vi "GetTerms3.vi"(0 "XRef":T10, 1 "State In":T9) -> (14 "Terms":T1)   [LabVIEW 2012, in "OpenG Search Array.xnode"]
doc: "This ability VI is used to describe your terminals to LabVIEW. Terms is an array of clusters describing the XNode's terminals.\n ID: A unique string identifying the terminal.\n Name: The name of the terminal visible to the user. Remember to localize it.\n Type: The data type of the terminal (as a Variant). The data put in the variant will be used as the default for the input terminal if it's left unwired.\n Bounds: A rectangle defining the bounds of the terminal relative to the bounds of the XNode. The bounds must be within the bounds of the XNode, and for whiskers to draw properly, they must be flush with at least one side of the XNode.\n Input?: Indicates whether or not this terminals is an input.\n Required?: Indicates whether the user must wire this terminal for the XNode to not be broken. Ignored on outputs.\n Recommended?: Indicates whether the terminal is recommended.\n Hidden?: Indicates whether the terminal is hidden. When a terminal is hidden, it cannot be wired to via user interaction or scripting. However, if it is already wired to when the hidden flag is changed to true, it will remain wired.\n Adaptive?: Indicates that the term should change to match the type of its source if it is wired.\n Direction?: Indicates what direction the wire stub should point. Choose auto to let LV decide based on the terms bounds being on the nodes edge.\n \n The IDs are used by LabVIEW to keep track of your terminals. When you respecify your terminals, LabVIEW can tell whther terminals are new, deleted, or moved by the unique IDs. The order is irrelevant. If you move a terminal, then any wire connected to it will move with it.\n \n If you want to update your terminals, you should return the UpdateTerms reply in one of your ability VIs.\n\nDefault behavior: None.\n\nThis ability does not provide UI and OS messages are not handled."
uses:
  OpenG Search Array.xnode
  <vilib>/XNodeSupport/XNodeXNodeRef.ctl
  State.ctl
  <vilib>/XNodeSupport/XNodeTerm3Array.ctl
  <vilib>/XNodeSupport/XNodeTerm3.ctl
  <vilib>/XNodeSupport/XNodeString.ctl
  <vilib>/XNodeSupport/XNodeVariant.ctl
  <vilib>/XNodeSupport/XNodeRect32.ctl
  <vilib>/XNodeSupport/XNodeInt.ctl
  <vilib>/XNodeSupport/XNodeBool.ctl
  <vilib>/XNodeSupport/XNodeTermDirection.ctl
  <vilib>/XNodeSupport/NI_XNodeSupport.lvlib
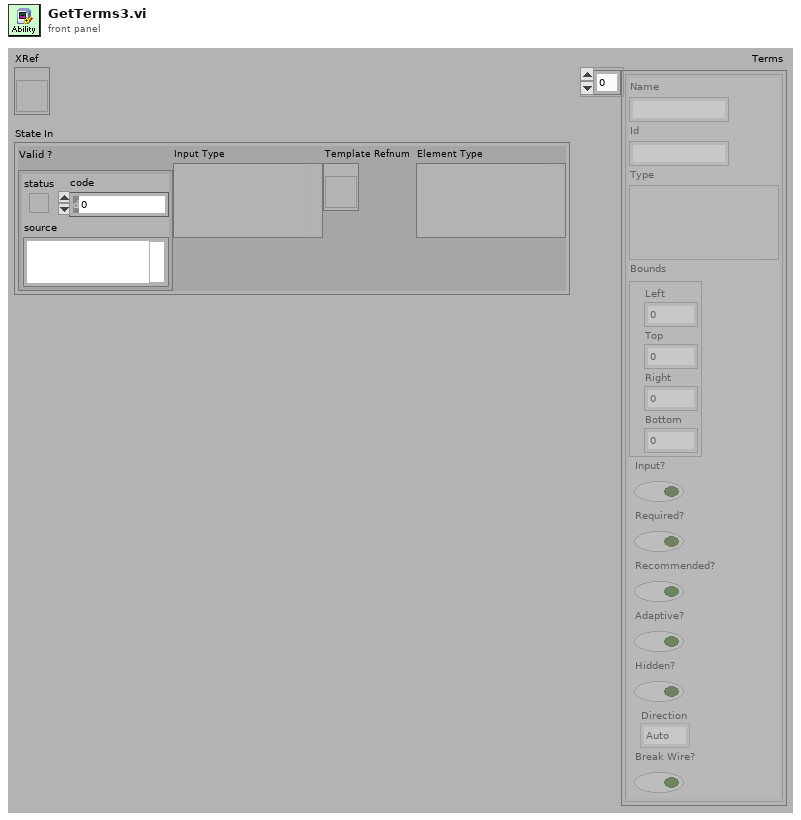
[diagram p1: front panel]
types:
  T1 = typedef "NI_XNodeSupport.lvlib/XNodeTerm3Array.ctl" = T2[]
  T2 = typedef "NI_XNodeSupport.lvlib/XNodeTerm3.ctl" = cluster{"Name":T3, "Id":T3, "Type":T4, "Bounds":T5, "Input?":T7, "Required?":T7, "Recommended?":T7, "Adaptive?":T7, "Hidden?":T7, "Direction":T8, "Break Wire?":T7}
  T3 = typedef "NI_XNodeSupport.lvlib/XNodeString.ctl" = string
  T4 = typedef "NI_XNodeSupport.lvlib/XNodeVariant.ctl" = variant
  T5 = typedef "NI_XNodeSupport.lvlib/XNodeRect32.ctl" = cluster{"Left":T6, "Top":T6, "Right":T6, "Bottom":T6}
  T6 = typedef "NI_XNodeSupport.lvlib/XNodeInt.ctl" = i32
  T7 = typedef "NI_XNodeSupport.lvlib/XNodeBool.ctl" = bool
  T8 = typedef "NI_XNodeSupport.lvlib/XNodeTermDirection.ctl" = enum32{"Auto", "Up", "Down", "Left", "Right", "Center"}
  T9 = typedef "OpenG Search Array.xnode/State.ctl" = cluster{"Valid ?":errorcluster, "Input Type":variant, "Template Refnum":refnum<vi>, "Element Type":variant}
  T10 = typedef "NI_XNodeSupport.lvlib/XNodeXNodeRef.ctl" = refnum<vi>
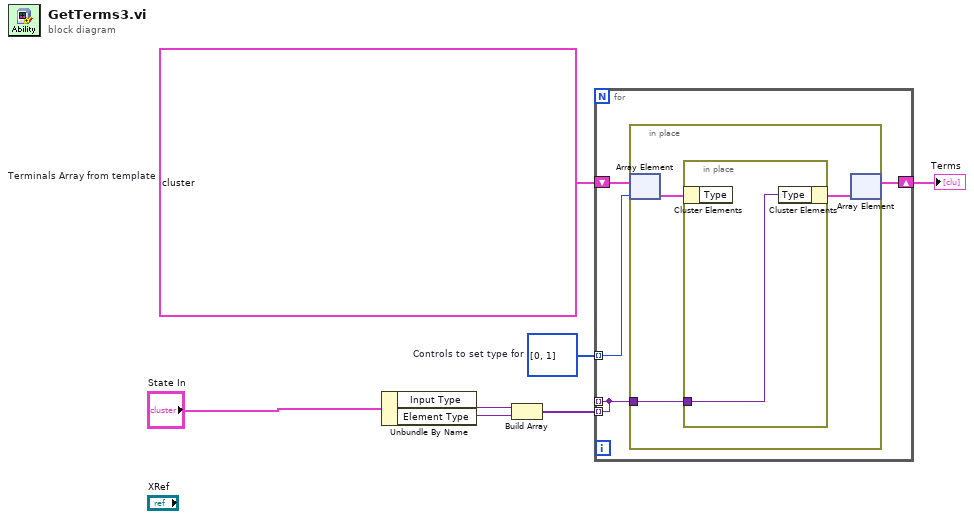
[diagram p0: block diagram]
diagram:
  w6 = i32[] [0, 1]  # Controls to set type for
  w7 = T2[] [{"Name"="Array", "Id"="0", "Type"=variant(i32[] []), "Bounds"={"Left"=0, "Top"=0, "Right"=8, "Bottom"=11}, "Input?"=TRUE, "Required?"=TRUE, "Recommended?"=TRUE, "Adaptive?"=FALSE, "Hidden?"=FALSE, "Direction"=enum."Auto", "Break Wire?"=FALSE}, {"Name"="Element Data", "Id"="2", "Type"=variant(i32 0), "Bounds"={"Left"=0, "Top"=11, "Right"=16, "Bottom"=21}, "Input?"=TRUE, "Required?"=TRUE, "Recommended?"=TRUE, "Adaptive?"=FALSE, "Hidden?"=FALSE, "Direction"=enum."Auto", "Break Wire?"=FALSE}, {"Name"="Start Index (0)", "Id"="3", "Type"=variant(i32 0), "Bounds"={"Left"=0, "Top"=21, "Right"=8, "Bottom"=32}, "Input?"=TRUE, "Required?"=FALSE, "Recommended?"=TRUE, "Adaptive?"=FALSE, "Hidden?"=FALSE, "Direction"=enum."Auto", "Break Wire?"=FALSE}, {"Name"="Indices of Elements", "Id"="7", "Type"=variant(i32[] []), "Bounds"={"Left"=16, "Top"=11, "Right"=32, "Bottom"=21}, "Input?"=FALSE, "Required?"=FALSE, "Recommended?"=TRUE, "Adaptive?"=FALSE, "Hidden?"=FALSE, "Direction"=enum."Auto", "Break Wire?"=FALSE}]  # Terminals Array from template
  n1 = Unbundle By Name("State In") -> ("Input Type"=w3:variant, "Element Type"=w2:variant)
  n2 = Build Array(w3, w2) -> (w1:variant[])
  n3 = for {
    tunnel: [w8] -> _ mode=indexing
    shift-right: [w10] -> w5
    shift-left: w7 -> [w11]
    tunnel: w6 -> [w9] mode=indexing
    tunnel: w1 -> [w8] mode=indexing
    n4 = in-place {
      in-place-border: w8 -> [w13]
      n5 = in-place-array #1(w11, w9) -> (w14:T2)
      n6 = in-place {
        in-place-border: w13 -> [w15]
        n7 = in-place-cluster #2(w14) -> ()  [unwired: 1 out]
        n8 = in-place-cluster #2("Type"=w15) -> (w12:T2)
      }
      n9 = in-place-array #1(w12) -> (w10:T2[])  [unwired: 1 out]
    }
  }
  "Terms" <- w5
